vi "getSenMfromFile.vi"(8 "error in":errorcluster, 10 "Sensitivity Matrix Shape":T1={"Num of Field"=35, "Num of Zk"=19, "Num of DOF"=50}, 11 "Path":path=path "/home/ttsai/Documents/stash/ts_tcs_ofc/configData/lsst/senM_35_19_50.txt") -> (0 "error out":errorcluster, 3 "Sensitivity Matrix":dbl[][][](array[numeric]))   [LabVIEW 2016]
doc: "Get the sensitivity matrix M from txt file."
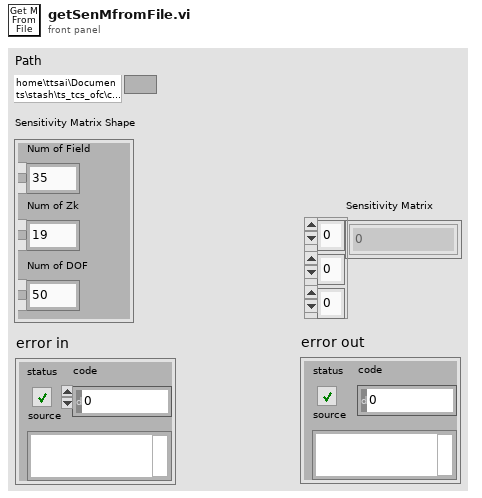
[diagram p1: front panel]
types:
  T1 = cluster{"Num of Field":i32, "Num of Zk":i32, "Num of DOF":i32}
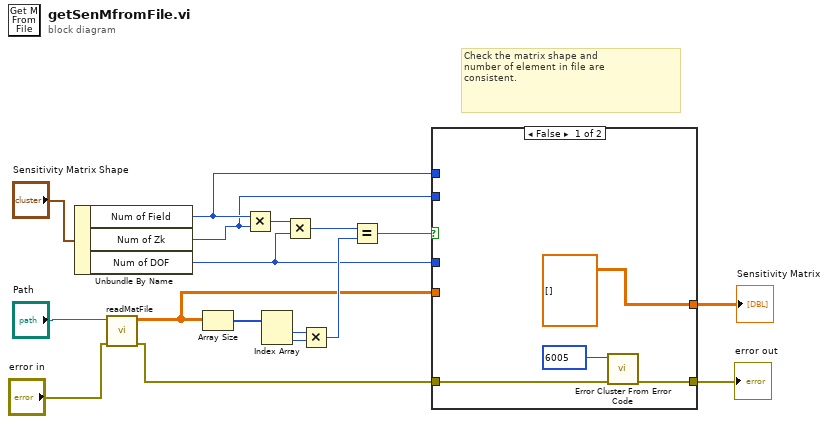
[diagram p0: block diagram]
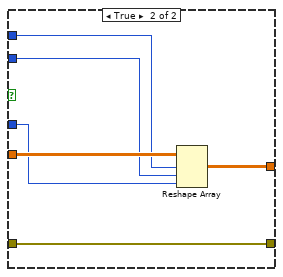
[diagram p2: hidden frame]
diagram:
  # "Check the matrix shape and \nnumber of element in file are\nconsistent."
  n1 = Unbundle By Name("Sensitivity Matrix Shape") -> ("Num of Field"=w4:i32, "Num of Zk"=w3:i32, "Num of DOF"=w2:i32)
  n2 = call "readMatFile.vi"("error in (no error)"="error in", "Path"="Path") -> ("error out"=w7:errorcluster, "Matrix"=w5:dbl[][])  [unwired: 8 in]
  n3 = Array Size(array=w5) -> (size(s)=w13:i32[])
  n4 = Multiply(x=w4, y=w3) -> (x*y=w14:i32)
  n5 = Index Array(array=w13) -> (element #1=w12:i32, element #2=w11:i32)  [unwired: 2 in]
  n6 = Multiply(x=w14, y=w2) -> (x*y=w9:i32)
  n7 = Multiply(x=w12, y=w11) -> (x*y=w10:i32)
  n8 = Equal?(x=w9, y=w10) -> (x = y?=w8:bool)
  n9 = case shown="False" w8 {
    tunnel: w7 -> [w20 w22]
    tunnel: [w19 w22] -> w6
    tunnel: w5 -> [_ w27]
    tunnel: w4 -> [_ w26]
    tunnel: w3 -> [_ w25]
    tunnel: w2 -> [_ w24]
    tunnel: [dbl[][][] [] ("Matrix") w23] -> w1
    frame False {
      n10 = call <vilib>:"Error Cluster From Error Code.vi"("error in (no error)"=w20, "error code (0)"=6005 ("code")) -> ("error out"=w19:errorcluster)  [unwired: 7 in]
    }
    frame True {
      n11 = Reshape Array(w27, w26, w25, w24) -> (w23:dbl[][][])
    }
  }
  "error out" <- w6
  "Sensitivity Matrix" <- w1
